vi "Initialize System Definition Tree.vi"(8 "error in":errorcluster, 11 "Item Ref in":T1 format="%.0x") -> (0 "error out":errorcluster, 3 "Item Ref out":T1 format="%.0x")   [LabVIEW 2019, in "HLA Custom Device System Explorer.lvlib"]
uses:
  HLA Custom Device System Explorer.lvlib
  <vilib>/NI VeriStand/Custom Device API/Custom Device Item Ref.ctl
  <vilib>/NI VeriStand/Custom Device API/Custom Device API.lvlib
  Shared/Constants.vi
  Shared/HLA Custom Device Shared.lvlib
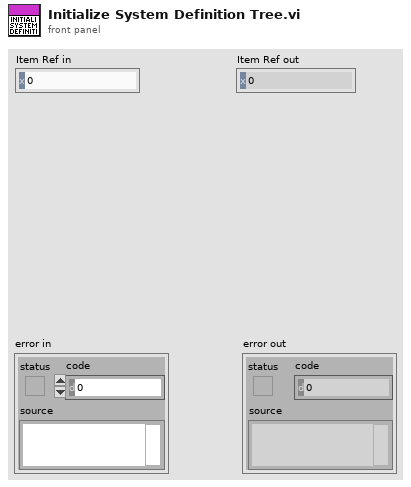
[diagram p1: front panel]
types:
  T1 = typedef "Custom Device API.lvlib/Custom Device Item Ref.ctl" = u64
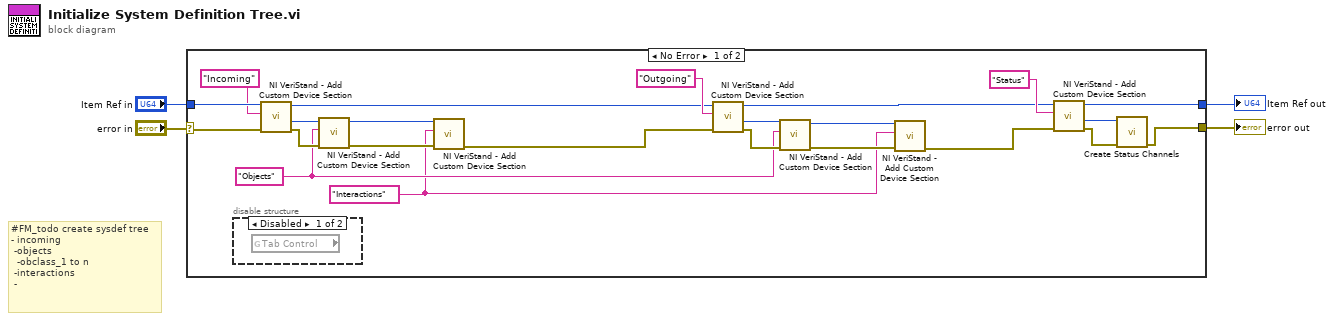
[diagram p0: block diagram]
diagram:
  # "#FM_todo create sysdef tree\n- incoming\n -objects\n  -obclass_1 to n\n -interactions\n -"
  n1 = case shown="No Error" "error in" {
    selector: "error in" -> [w26 w28]
    tunnel: "Item Ref in" -> [w27 w29]
    tunnel: [w9 w29] -> w2
    tunnel: [w5 w28] -> w1
    frame No Error {
      w12 = "Interactions" ("Section Name")
      w13 = "Objects" ("Section Name")
      n2 = disable-structure shown="Disabled" {
        frame Disabled {
          n3 = global read "Constants.vi" "Tab Control"() -> ()  [unwired: 1 out]
        }
        frame Enabled {
        }
      }
      n4 = call <vilib>:"NI VeriStand - Add Custom Device Section.vi"("error in (no error)"=w26, "Section Name"="Incoming", "Parent Ref in"=w27) -> ("error out"=w21:errorcluster, "Section Ptr"=w22:T1, "Parent Ref out"=w23:T1)  [unwired: 5 in, 1 out]
      n5 = call <vilib>:"NI VeriStand - Add Custom Device Section.vi"("error in (no error)"=w21, "Section Name"=w13, "Parent Ref in"=w22) -> ("error out"=w20:errorcluster, "Parent Ref out"=w19:T1)  [unwired: 5 in, 2 out]
      n6 = call <vilib>:"NI VeriStand - Add Custom Device Section.vi"("error in (no error)"=w20, "Section Name"=w12, "Parent Ref in"=w19) -> ("error out"=w18:errorcluster)  [unwired: 5 in, 3 out]
      n7 = call <vilib>:"NI VeriStand - Add Custom Device Section.vi"("error in (no error)"=w18, "Section Name"="Outgoing", "Parent Ref in"=w23) -> ("error out"=w15:errorcluster, "Section Ptr"=w14:T1, "Parent Ref out"=w10:T1)  [unwired: 5 in, 1 out]
      n8 = call <vilib>:"NI VeriStand - Add Custom Device Section.vi"("error in (no error)"=w15, "Section Name"=w13, "Parent Ref in"=w14) -> ("error out"=w16:errorcluster, "Parent Ref out"=w17:T1)  [unwired: 5 in, 2 out]
      n9 = call <vilib>:"NI VeriStand - Add Custom Device Section.vi"("error in (no error)"=w16, "Section Name"=w12, "Parent Ref in"=w17) -> ("error out"=w8:errorcluster)  [unwired: 5 in, 3 out]
      n10 = call <vilib>:"NI VeriStand - Add Custom Device Section.vi"("error in (no error)"=w8, "Section Name"="Status", "Parent Ref in"=w10) -> ("error out"=w7:errorcluster, "Section Ptr"=w6:T1, "Parent Ref out"=w9:T1)  [unwired: 5 in, 1 out]
      n11 = call "Create Status Channels.vi"("error in"=w7, "Device Item Ref in"=w6) -> ("error out"=w5:errorcluster)  [unwired: 8 in, 1 out]
    }
    frame Error {
    }
  }
  "error out" <- w1
  "Item Ref out" <- w2
